vi "GetResolution.vi"(8 "error in (no error)":errorcluster, 11 "CameraTesting in":refnum<class "CameraTesting.lvclass">) -> (0 "error out":errorcluster, 3 "CameraTesting out":refnum<class "CameraTesting.lvclass">)   [LabVIEW 2020, in "CameraTesting.lvlib" / "CameraTesting.lvclass"]
uses:
  CameraTesting.lvclass
  CameraTesting.lvclass/CameraTesting.ctl
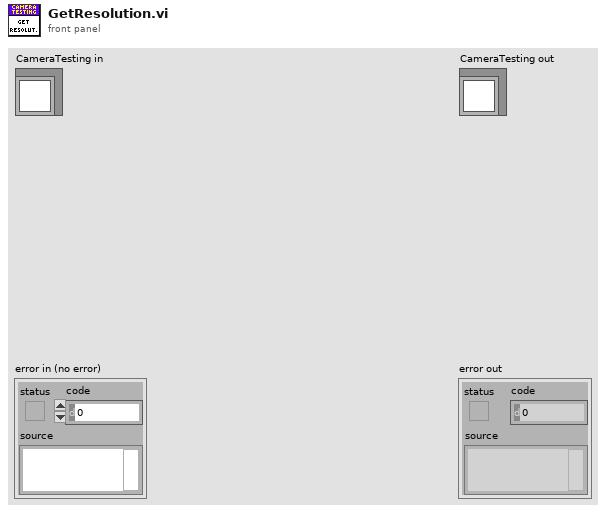
[diagram p1: front panel]
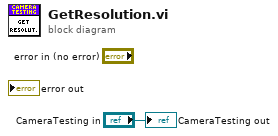
[diagram p0: block diagram]
diagram:
  "CameraTesting out" <- "CameraTesting in"
